vi "Get Result as Date.vi"(8 "error in (no error)":errorcluster, 11 "Parameter in":refnum<class "Parameter.lvclass">) -> (0 "error out":errorcluster, 2 "Result":timestamp format="%<%d/%m/%Y>T", 3 "Parameter out":refnum<class "Parameter.lvclass">)   [LabVIEW 2023, in "HAF.lvlib" / "Parameter.lvclass"]
doc: "Returns the raw result as a Date only Timestamp. Time defaults to midnight. If the raw result is not compatible, then an error is raised."
uses:
  Parameter.lvclass
  Parameter.lvclass/Parameter.ctl
  HAF.lvlib
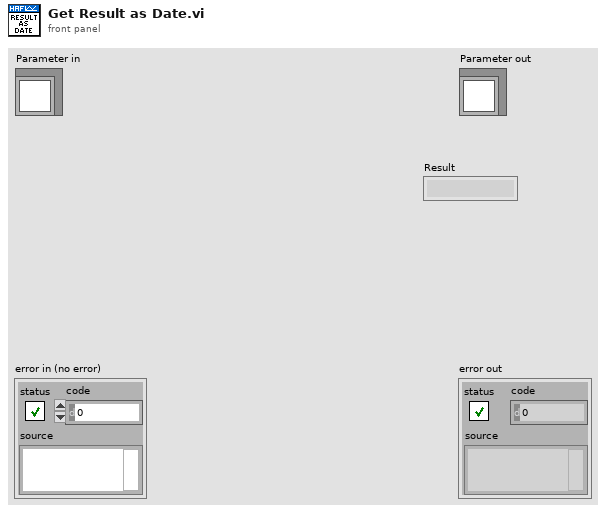
[diagram p1: front panel]
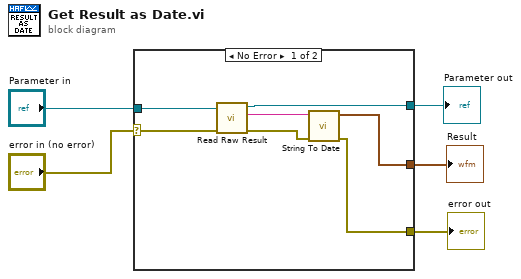
[diagram p0: block diagram]
diagram:
  n1 = case shown="No Error" "error in (no error)" {
    selector: "error in (no error)" -> [w11 w14]
    tunnel: [w6 w14] -> w4
    tunnel: [w8 w13] -> w2
    tunnel: "Parameter in" -> [w12 w13]
    tunnel: [w7 _] -> w1
    frame No Error {
      n2 = call-dynamic "Read Raw Result.vi"("error in (no error)"=w11, "Parameter in"=w12) -> ("error out"=w9:errorcluster, "Raw Result"=w10:string, "Parameter out"=w8:refnum<class "Parameter.lvclass">)  [unwired: 7 in]
      n3 = call "String To Date.vi"("error in (no error)"=w9, "String to Convert"=w10) -> ("error out"=w6:errorcluster, "Date Value"=w7:timestamp)  [unwired: 8 in]
    }
    frame Error {
    }
  }
  "error out" <- w4
  "Parameter out" <- w2
  "Result" <- w1
